vi "I2C_Read_1_Bit_DAQ.vi"() -> (2 "RX_Bit_Out":bool)   [LabVIEW 2022 SP3]
doc: "Petrus Prins 7 June 2026"
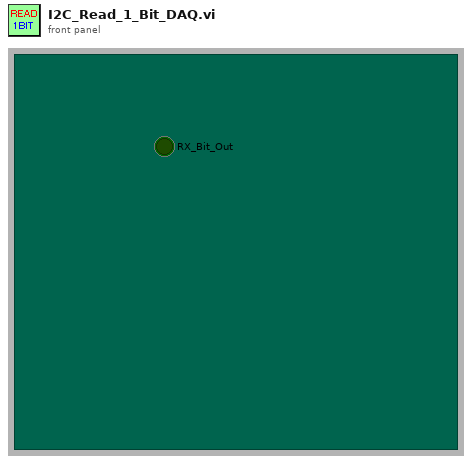
[diagram p1: front panel]
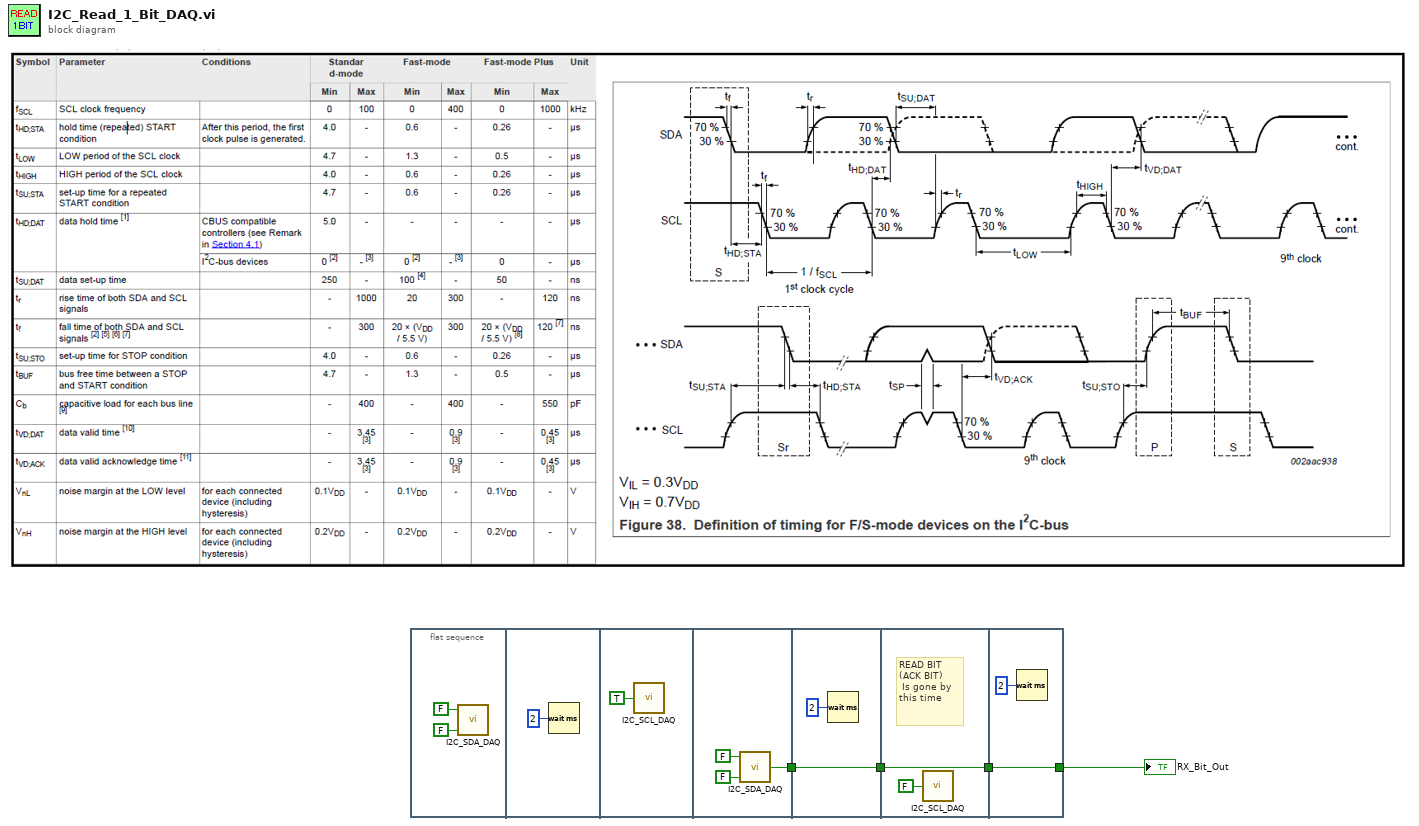
[diagram p0: block diagram]
diagram:
  n1 = flat-sequence {
    tunnel: [w9] -> w3
    tunnel: w3 -> [w13]
    tunnel: [w13] -> w2
    tunnel: w2 -> [w15]
    tunnel: [w15] -> w1
    tunnel: [w17] -> w4
    tunnel: w1 -> [w17]
    frame #0 {
      n2 = call "I2C_SDA_DAQ.vi"("Tx_or_Rx?"=FALSE, "Tx_Data"=FALSE) -> ()  [unwired: 1 in, 1 out]
    }
    frame #1 {
      n3 = Wait (ms)(milliseconds to wait=u32 2) -> ()  [unwired: 1 out]
    }
    frame #2 {
      n4 = call "I2C_SCL_DAQ.vi"("SCL_Data"=TRUE) -> ()  [unwired: 5 in]
    }
    frame #3 {
      n5 = call "I2C_SDA_DAQ.vi"("Tx_or_Rx?"=FALSE, "Tx_Data"=FALSE) -> ("Rx_Data"=w9:bool)  [unwired: 1 in]
    }
    frame #4 {
      n6 = Wait (ms)(milliseconds to wait=u32 2) -> ()  [unwired: 1 out]
    }
    frame #5 {
      # "READ BIT (ACK BIT)\n Is gone by this time"
      n7 = call "I2C_SCL_DAQ.vi"("SCL_Data"=FALSE) -> ()  [unwired: 5 in]
    }
    frame #6 {
      n8 = Wait (ms)(milliseconds to wait=u32 2) -> ()  [unwired: 1 out]
    }
  }
  "RX_Bit_Out" <- w4
